vi "Test.vi"(8 "error in (no error)":errorcluster, 10 "board image":T1, 11 "Elite DAQ Design in":refnum<class "Elite DAQ Design.lvclass">) -> (0 "error out":errorcluster, 2 "pass?":T2, 3 "Test name":string)   [LabVIEW 2018, in "Elite DAQ Design.lvclass"]
doc: "Image check for blocks that are common to this board type."
uses:
  Elite DAQ Design.lvclass
  Common/Pass Fail Boolean.ctl
  Common/Board Image.ctl
  DAQ Board Design_class/DAQ Board Design.lvclass
  Board Design_class/Board Design.lvclass
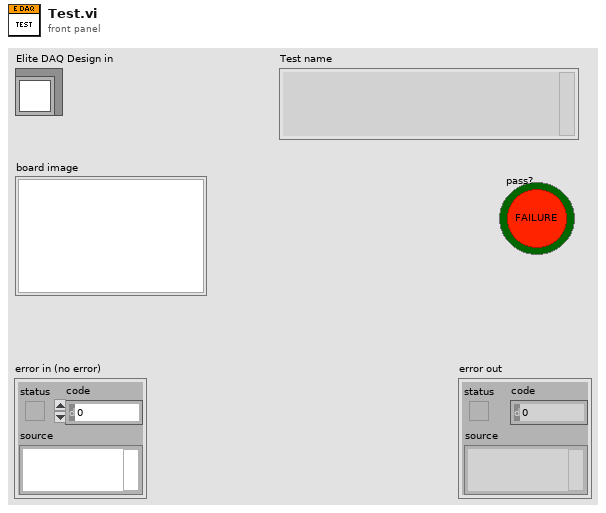
[diagram p1: front panel]
types:
  T1 = typedef "Board Image.ctl" = picture
  T2 = typedef "Pass Fail Boolean.ctl" = bool
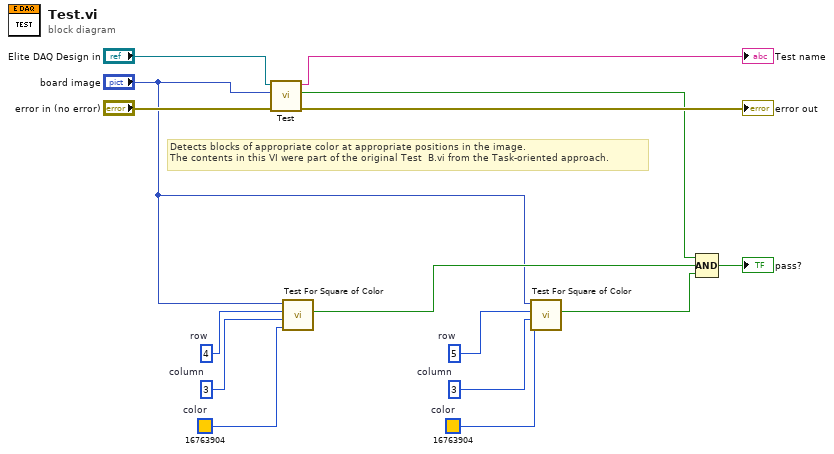
[diagram p0: block diagram]
diagram:
  w7 = i16 3  # column
  w6 = i16 5  # row
  w8 = u32 16763904  # color
  w10 = i16 3  # column
  w11 = i16 4  # row
  w9 = u32 16763904  # color
  # "Detects blocks of appropriate color at appropriate positions in the image.\nThe contents in this VI were part of the original Test  B.vi from the Task-oriented approach."
  n1 = call-parent "Test.vi"("error in (no error)"="error in (no error)", "board image"="board image", "DAQ Board Design in"="Elite DAQ Design in") -> ("error out"=→"error out":errorcluster, "pass?"=w2:T2, "Test name"=→"Test name":string)  [unwired: 6 in]
  n2 = call "Test For Square of Color.vi"("color"=w9, "column"=w10, "row"=w11, "board image"="board image") -> ("pass?"=w5:T2)  [unwired: 7 in]
  n3 = call "Test For Square of Color.vi"("color"=w8, "column"=w7, "row"=w6, "board image"="board image") -> ("pass?"=w4:T2)  [unwired: 7 in]
  n4 = Compound Arithmetic op=AND(w2, w5, w4) -> (→"pass?":T2)
